vi "Get pulse count.vi"() -> (0 "Error":errorcluster, 1 "Sample DateTime":timestamp, 2 "Pulse count":u32)   [LabVIEW 2011]
uses:
  <vilib>/DAQmx/read.llb/DAQmx Read (Counter U32 1Chan 1Samp).vi
  <vilib>/DAQmx/miscellaneous.llb/DAQmx Fill In Error Info.vi
panel:
  # "by Paul Nathan, 01/03/2012"
  # "Revisions:\nDate       Desc.      Auth.\nx               x               x"
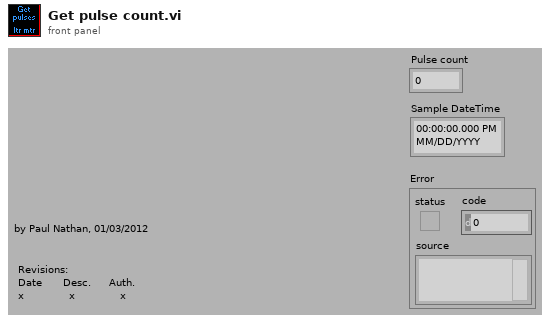
[diagram p1: front panel]
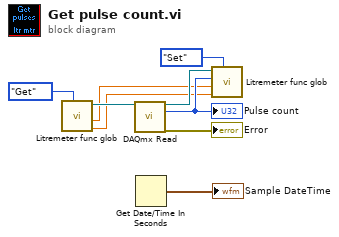
[diagram p0: block diagram]
diagram:
  n1 = call "Litremeter func glob.vi"("Action"=enum16{"Get", "Set"}."Get") -> ("Offset Litres out"=w2:dbl, "Litres / pulse out"=w1:dbl, "Counter task out"=w6:refnum<k21>)  [unwired: 4 in, 2 out]
  n2 = call-poly <vilib>:"DAQmx Read.vi"("task/channels in"=w6) -> ("task out"=w4:refnum<k21>, "data"=w3:u32, "error out"=→"Error":errorcluster)  [unwired: 12 in]
  "Pulse count" <- w3
  n3 = Get Date/Time In Seconds() -> (seconds since 1Jan1904=→"Sample DateTime":timestamp)
  n4 = call "Litremeter func glob.vi"("Action"=enum16{"Get", "Set"}."Set", "Offset Litres in"=w2, "Litres / pulse in"=w1, "Pulse count in"=w3, "Counter task in"=w4) -> ()  [unwired: 5 out]
